vi "Log Message.vi"(8 "error constant":errorcluster, 10 "input":string) -> (0 "error constant 2":errorcluster, 2 "output":string)   [LabVIEW 2023]
uses:
  GLOBAL/GLOBAL Debug.vi
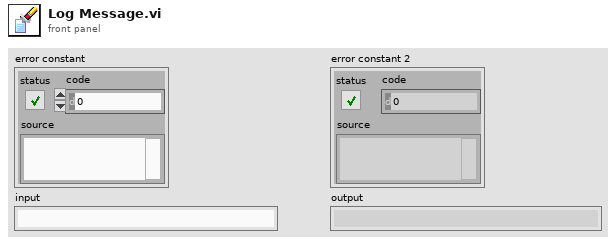
[diagram p1: front panel]
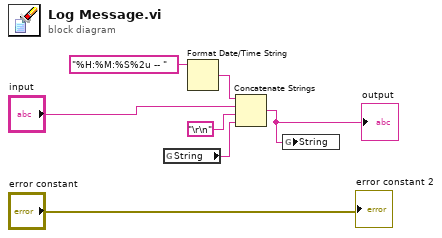
[diagram p0: block diagram]
diagram:
  n1 = global read "GLOBAL Debug.vi" "String"() -> (w4:string)
  n2 = Format Date/Time String(time format string (%c)="%H:%M:%S%2u -- ") -> (date/time string=w2:string)  [unwired: 2 in]
  n3 = Concatenate Strings(w2, "input", "\r\n", w4) -> (w3:string)
  "output" <- w3
  n4 = global write "GLOBAL Debug.vi" "String"(w3) -> ()
  "error constant 2" <- "error constant"
